vi "Data Type to U32.vi"(8 "error in (no error)":errorcluster, 11 "Data Type":refnum<class "Data Type.lvclass">) -> (0 "error out":errorcluster, 3 "U32 out":u32)   [LabVIEW 2017, in "U32.lvclass"]
uses:
  <vilib>/gpm_packages/@cs/data-type-serializer/source/U32/U32.lvclass
  <vilib>/gpm_packages/@cs/data-type-serializer/source/Data Type/Data Type.lvclass
  <vilib>/gpm_packages/@cs/data-type-serializer/source/U32/U32.lvclass/U32.ctl
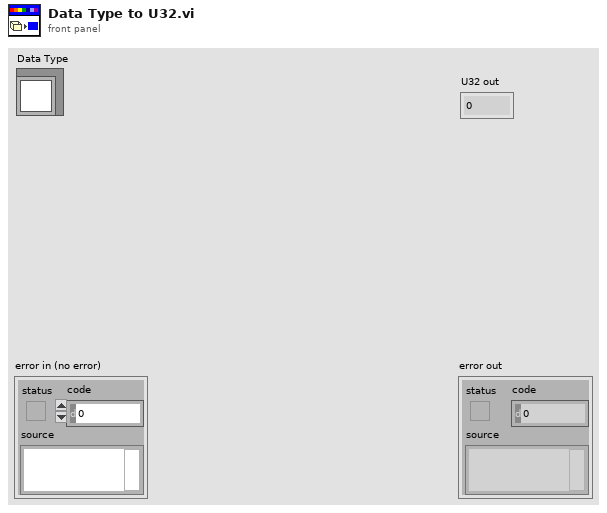
[diagram p1: front panel]
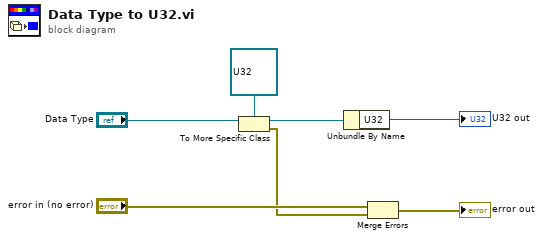
[diagram p0: block diagram]
diagram:
  n1 = To More Specific Class(target class=refnum<class "U32.lvclass"> refnum ("Boolean out"), reference="Data Type") -> (specific class reference=w4:refnum<class "U32.lvclass">, error out=w1:errorcluster)  [unwired: 1 in]
  n2 = Unbundle By Name(w4) -> ("U32"=→"U32 out":u32)
  n3 = Merge Errors("error in (no error)", w1) -> (→"error out":errorcluster)
